vi "create log file.vi"(8 "error in":errorcluster, 11 "Cluster in":T1={"This VI Ref"=refnum, "Test VI"=refnum, "Q Ref"=refnum, "UE"=refnum, "Data"=variant, "Timeout"=-1, "Path List[]"=[], "Status"="", "Counter"=0, "Config"={"Source Path"=path "", "Dest Path"=path "", "Log Path"=path "", "Move?"=FALSE, "Log?"=FALSE, "Scanners"=[], "Excude Folders"=[], "Jpg?"=FALSE, "Default path"=path "", "Extended?"=FALSE, "Mode"=enum."Move"}, "Total"=0, "Config Path"=path "", "exif info"={"Make"="Canon\u0000", "Model"="Canon PowerShot A495\u0000", "Orientation"=0, "Date"=timestamp(0 s since 1904-01-01), "Width"=0, "Height"=0, "Square?"=FALSE, "File Name"="Canon\u0000", "Extension"="Canon\u0000", "Valid?"=FALSE, "Path"=path "", "size"=0, "No Ext?"=FALSE, "prefix?"=FALSE, "String"="", "Name Type"=enum."Event Sufix"}, "app operation"=enum."Start", "Log Ref"=refnum, "Start Time"=0.0, "Pause Time"=0.0, "Argument?"=FALSE, "Argument path"=path "", "Identical"=FALSE, "File.lvclass"=refnum}) -> (0 "error out":errorcluster, 3 "Cluster out":T1={"This VI Ref"=refnum, "Test VI"=refnum, "Q Ref"=refnum, "UE"=refnum, "Data"=variant, "Timeout"=-1, "Path List[]"=[], "Status"="", "Counter"=0, "Config"={"Source Path"=path "", "Dest Path"=path "", "Log Path"=path "", "Move?"=FALSE, "Log?"=FALSE, "Scanners"=[], "Excude Folders"=[], "Jpg?"=FALSE, "Default path"=path "", "Extended?"=FALSE, "Mode"=enum."Move"}, "Total"=0, "Config Path"=path "", "exif info"={"Make"="Canon\u0000", "Model"="Canon PowerShot A495\u0000", "Orientation"=0, "Date"=timestamp(0 s since 1904-01-01), "Width"=0, "Height"=0, "Square?"=FALSE, "File Name"="Canon\u0000", "Extension"="Canon\u0000", "Valid?"=FALSE, "Path"=path "", "size"=0, "No Ext?"=FALSE, "prefix?"=FALSE, "String"="", "Name Type"=enum."Event Sufix"}, "app operation"=enum."Start", "Log Ref"=refnum, "Start Time"=0.0, "Pause Time"=0.0, "Argument?"=FALSE, "Argument path"=path "", "Identical"=FALSE, "File.lvclass"=refnum})   [LabVIEW 2023, in "User Interface.lvlib"]
uses:
  User Interface.lvlib
  Controls/main consumer cluster.ctl
  File Classes/File/File.lvclass
  Controls/configuration cluster.ctl
  File Classes/Controls/exif data cluster.ctl
  File Classes/Controls/rename type enum.ctl
  Controls/app operation state enum.ctl
  <vilib>/Utility/sysdir.llb/System Directory Type.ctl
  File Classes/File Classes.lvlib
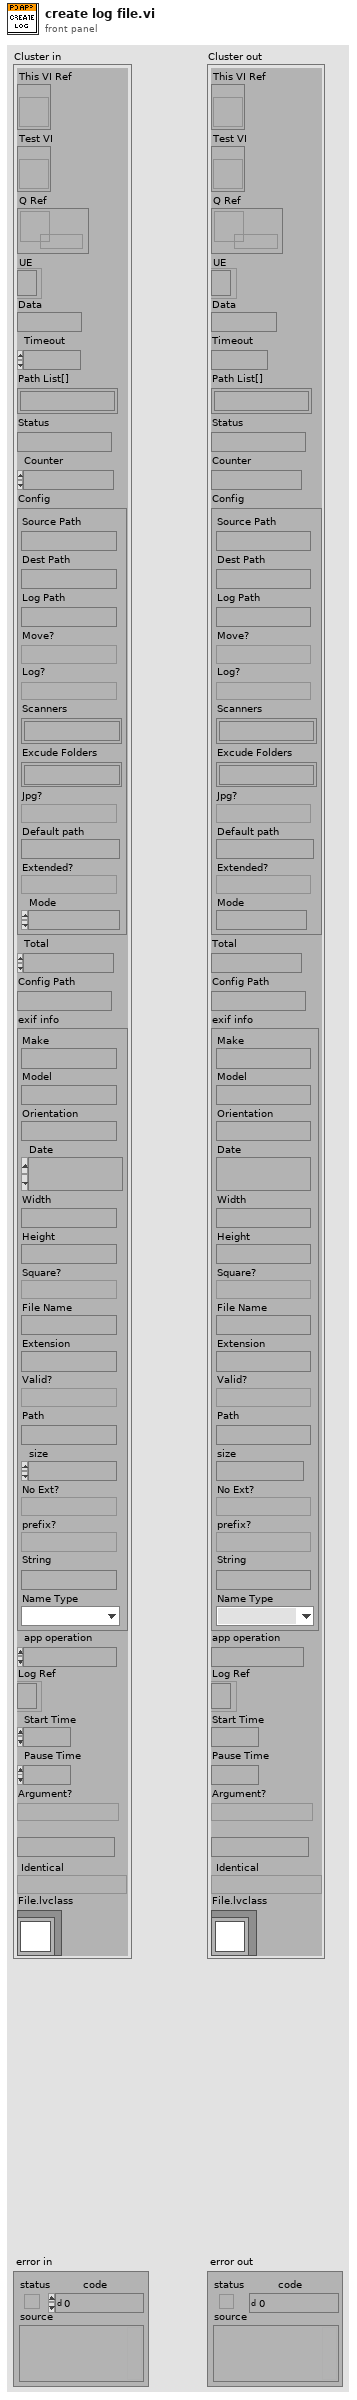
[diagram p1: front panel]
types:
  T1 = typedef "User Interface.lvlib/main consumer cluster.ctl" = cluster{"This VI Ref":refnum<vi>, "Test VI":refnum<vi>, "Q Ref":refnum<queue>, "UE":refnum<event-registration>, "Data":variant, "Timeout":i32, "Path List[]":path[], "Status":string, "Counter":i32, "Config":T2, "Total":i32, "Config Path":path, "exif info":T3, "app operation":T5, "Log Ref":refnum<file>, "Start Time":dbl, "Pause Time":dbl, "Argument?":bool, "Argument path":path, "Identical":bool, "File.lvclass":refnum<class "File.lvclass">}
  T2 = typedef "User Interface.lvlib/configuration cluster.ctl" = cluster{"Source Path":path, "Dest Path":path, "Log Path":path, "Move?":bool, "Log?":bool, "Scanners":string[], "Excude Folders":string[], "Jpg?":bool, "Default path":path, "Extended?":bool, "Mode":enum16{"Copy (Default)", "Move", "Rename"}}
  T3 = typedef "File Classes.lvlib/exif data cluster.ctl" = cluster{"Make":string, "Model":string, "Orientation":u16, "Date":timestamp, "Width":u16, "Height":u16, "Square?":bool, "File Name":string, "Extension":string, "Valid?":bool, "Path":path, "size":i64, "No Ext?":bool, "prefix?":bool, "String":string, "Name Type":T4}
  T4 = typedef "File Classes.lvlib/rename type enum.ctl" = enum16{"Date & Time (Default)", "Model Sufix", "Event Sufix", "Model & Event Sufix"}
  T5 = typedef "User Interface.lvlib/app operation state enum.ctl" = enum16{"Start", "Stop", "Pause", "Resume"}
  T6 = enum16{"open", "replace", "create", "open or create", "replace or create", "replace or create with confirmation"}
  T7 = typedef "System Directory Type.ctl" = i32
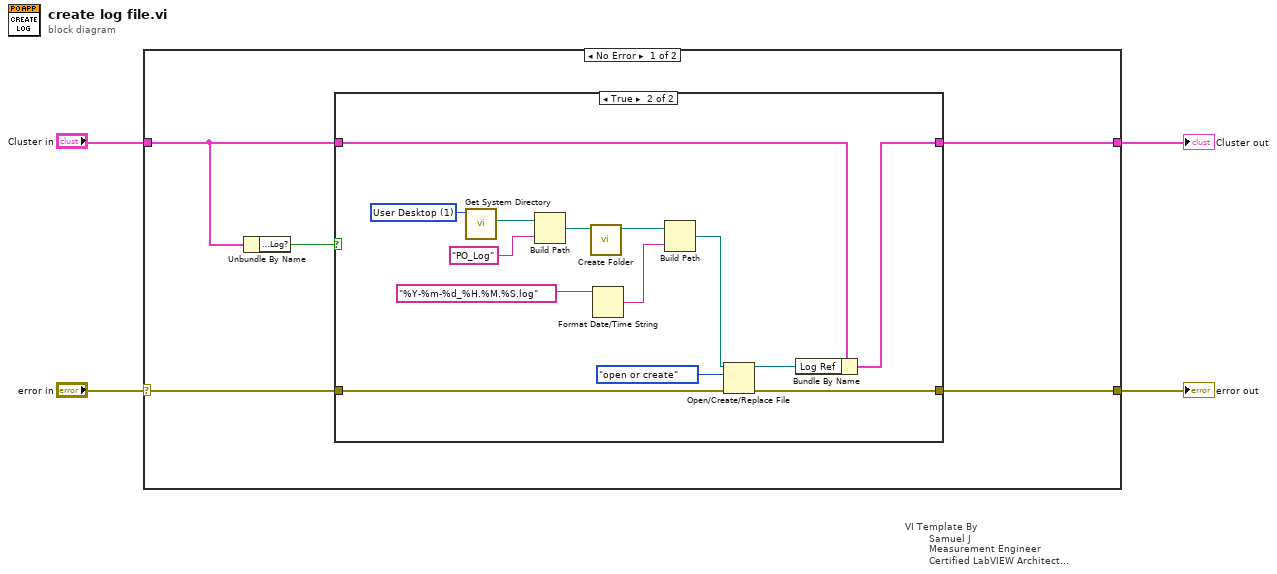
[diagram p0: block diagram]
diagram:
  n1 = case "VI Template By\n        Samuel J\n        Measurement Engineer\n        Certified LabVIEW Architect\n        Vestas Technology R&D Chennai" shown="No Error" "error in" {
    selector: "error in" -> [w6 w27]
    tunnel: [w5 w27] -> w3
    tunnel: [w7 w26] -> w2
    tunnel: "Cluster in" -> [w8 w26]
    frame No Error {
      n2 = Unbundle By Name(w8) -> ("Config.Log?"=w9:bool)
      n3 = case shown="True" w9 {
        tunnel: w6 -> [w10 w16]
        tunnel: [w10 w15] -> w5
        tunnel: w8 -> [w11 w14]
        tunnel: [w11 w13] -> w7
        frame False {
        }
        frame True {
          w25 = T7 1 items=["User Home"=0, "User Desktop"=1, "User Documents"=2, "User Application Data"=3, "User Preferences"=4, "User Temporary"=5, "Public Documents"=6, "Public Application Data"=7, "Public Preferences"=8, "Public Cache"=13, "System Core Libraries"=9, "System Installed Libraries"=10, "Application Files"=11, "Boot Volume Root"=12] ("system directory type")
          n4 = call <vilib>:"Get System Directory.vi"("system directory type"=w25) -> ("system directory"=w24:path)  [unwired: 10 in]
          n5 = Build Path(base path=w24, name or relative path="PO_Log") -> (appended path=w22:path)
          n6 = call <userlib>:"Create Folder.vi"("Directory Path"=w22) -> ("dup Directory Path"=w21:path)  [unwired: 9 in, 1 out]
          n7 = Format Date/Time String(time format string (%c)="%Y-%m-%d_%H.%M.%S.log") -> (date/time string=w19:string)  [unwired: 2 in]
          n8 = Build Path(base path=w21, name or relative path=w19) -> (appended path=w18:path)
          n9 = Open/Create/Replace File(file path (use dialog)=w18, error in=w16, operation (0:open)=T6."open or create") -> (refnum out=w12:refnum<file>, error out=w15:errorcluster)  [unwired: 3 in, 1 out]
          n10 = Bundle By Name(cluster=w14, "Log Ref"=w12) -> (w13:T1)
        }
      }
    }
    frame Error {
    }
  }
  "error out" <- w3
  "Cluster out" <- w2
